vi "Read Layout.vi"(11 "Log Sinks in":refnum<class "Log Sinks.lvclass">) -> (2 "Layout":refnum<class "Layout.lvclass">, 3 "Log Sinks out":refnum<class "Log Sinks.lvclass">)   [LabVIEW 2019, in "TSC Event Logger.lvlib" / "Log Sinks.lvclass"]
uses:
  Log Sinks.lvclass
  Layouts/Layout.lvclass
  Log Sinks.lvclass/Log Sinks.ctl
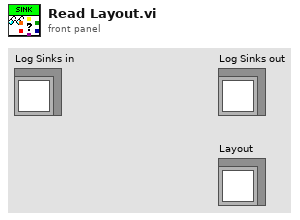
[diagram p1: front panel]
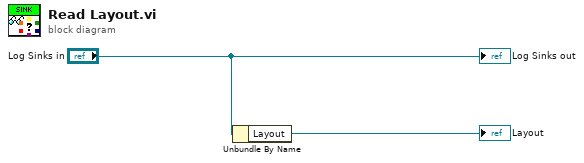
[diagram p0: block diagram]
diagram:
  n1 = Unbundle By Name("Log Sinks in") -> ("Layout"=→"Layout":refnum<class "Layout.lvclass">)
  "Log Sinks out" <- "Log Sinks in"
